vi "createTDMS.vi"(0 "path":path=path "C:/ni-rt/startup/datalog/temp", 1 "channel name(s)":string[](array[string])=["Time UTC", "I_src", "V_src", "BMS_Vbat", "BMS_Ibat", "BMS_SoC", "BMS_SoH"], 2 "file basename":string="battery_") -> (3 "Ref":refnum<k34>, 5 "hour":string, 6 "error out":errorcluster)   [LabVIEW 2021]
panel:
  in  "overwrite?":bool
  in  "error in":errorcluster
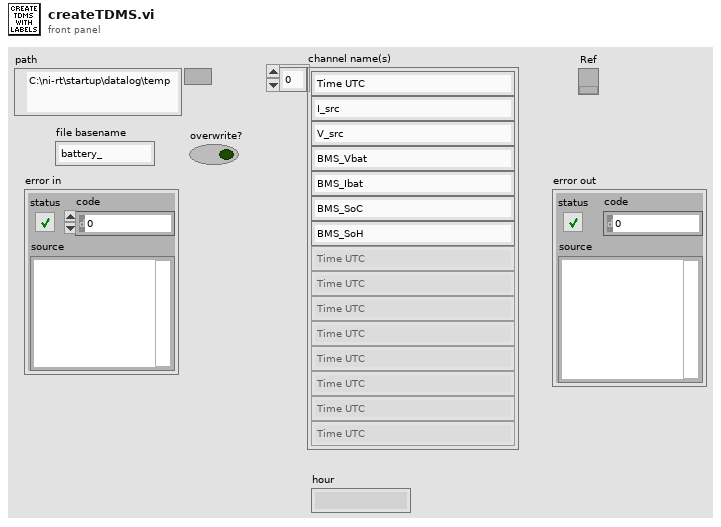
[diagram p1: front panel]
types:
  T1 = enum16{"open", "open or create", "create or replace", "create", "open (read-only)"}
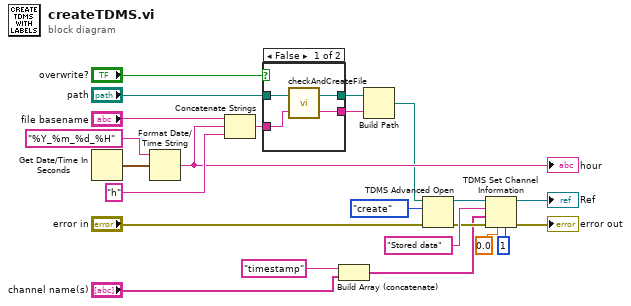
[diagram p0: block diagram]
diagram:
  n1 = Get Date/Time In Seconds() -> (seconds since 1Jan1904=w19:timestamp)
  n2 = Format Date/Time String(time format string (%c)="%Y_%m_%d_%H", seconds (now)=w19) -> (date/time string=w20:string)  [unwired: 1 in]
  "hour" <- w20
  n3 = Concatenate Strings("file basename", w20, "h" ("string")) -> (w9:string)
  n4 = case shown="False" "overwrite?" {
    tunnel: w9 -> [w27 w28]
    tunnel: "path" -> [w26 w29]
    tunnel: [w25 w29] -> w6
    tunnel: [w24 w28] -> w5
    frame False {
      n5 = call "checkAndCreateFile.vi"("filename"=w27, "path in"=w26) -> ("filename out"=w24:string, "path out"=w25:path)
    }
    frame True {
    }
  }
  n6 = Build Array (concatenate)("timestamp", "channel name(s)") -> (w2:string[])
  n7 = Build Path(base path=w6, name or relative path=w5) -> (appended path=w7:path)
  n8 = TDMS Advanced Open(8:"error in", 10:T1."create" ("operation (0:open)"), 11:w7) -> (0:w13:errorcluster, 3:w12:refnum<k34>)  [unwired: 2 in, 1 out]
  n9 = TDMS Set Channel Information(4:u32 1 ("samples per channel"), 6:0.0, 8:w13, 9:w2, 10:"Stored data" ("group name in (Untitled)"), 11:w12) -> (0:→"error out":errorcluster, 3:→"Ref":refnum<k34>)  [unwired: 1 in]
